vi "DAQmx Create Channel (TEDS-AI-Bridge).vi"(0 "task in":refnum<k21>, 1 "maximum value":dbl=0.002 format="%.3f", 2 "minimum value":dbl=-0.002 format="%.3f", 5 "physical channels":tag, 7 "name to assign":string, 9 "units":i32(ring)=12516 items=["From TEDS"=12516, "From Custom Scale"=10065], 11 "error in":errorcluster, 12 "custom scale name":tag, 13 "voltage excitation source":i32(ring)=10200 items=["Internal"=10200, "External"=10167], 14 "voltage excitation value":dbl=2.5) -> (4 "task out":refnum<k21>, 15 "error out":errorcluster)   [LabVIEW 2011]
doc: "Creates channel(s) that measure a Wheatstone bridge. You must configure the physical channel(s) with TEDS information to use this VI. Use this instance with bridge-based sensors that measure phenomena other than strain, force, pressure, or torque, or that scale data to physical units NI-DAQmx does not support."
uses:
  C:/Program Files/National Instruments/LabVIEW 2011/resource/objmgr/daqmx.rc
panel:
  # "input limits"
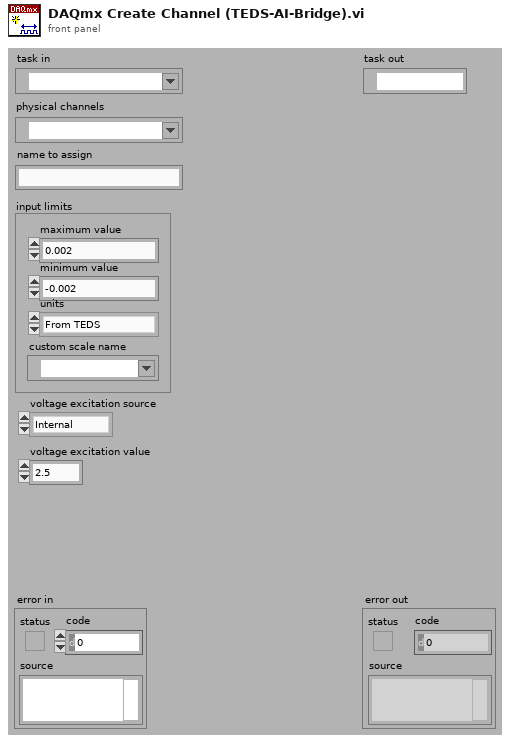
[diagram p1: front panel]
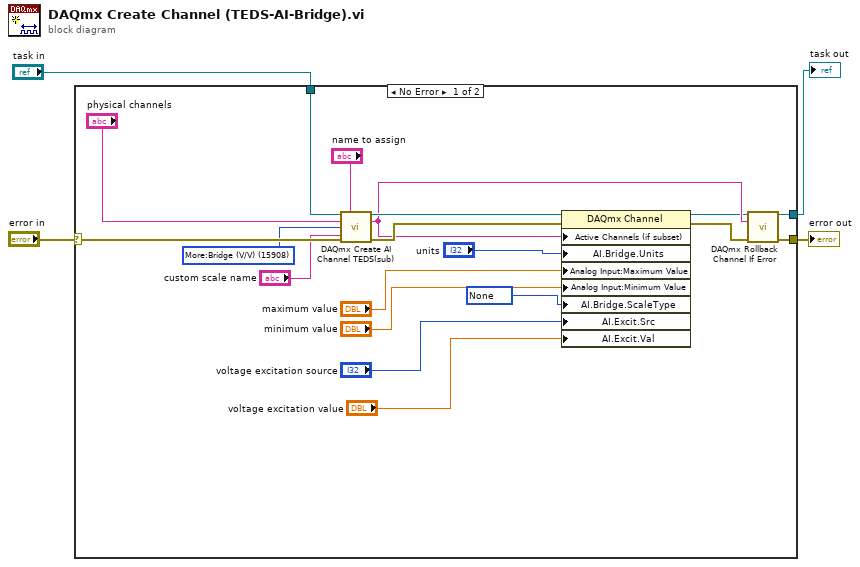
[diagram p0: block diagram]
diagram:
  n1 = case shown="No Error" "error in" {
    selector: "error in" -> [w22 w24]
    tunnel: [w14 w24] -> w4
    tunnel: "task in" -> [w23 w25]
    tunnel: [w13 w25] -> w1
    frame No Error {
      w8 = 10230 items=["None"=10230, "Two-Point Linear"=15898, "Table"=10450, "Polynomial"=10449] ("AI.Bridge.ScaleType")
      w9 = 15908 items=["Voltage"=10322, "Voltage RMS"=10350, "Current"=10134, "Current RMS"=10351, "More:Voltage:Custom with Excitation"=10323, "More:Bridge (V/V)"=15908, "Frequency"=10181, "Resistance"=10278, "Temperature:Thermocouple"=10303, "Temperature:Thermistor"=10302, "Temperature:RTD"=10301, "Temperature:Built-in Sensor"=10311, "Strain Gage"=10300, "Position:LVDT"=10352, "Position:RVDT"=10353, "Position:Eddy Current Proximity Probe"=14835, "Accelerometer"=10356, "Force:Bridge (Two-Point Linear)"=15899, "Force:Bridge (Table)"=15900, "Force:Bridge (Polynomial)"=15901, "Force:IEPE Sensor"=15895, "Pressure:Bridge (Two-Point Linear)"=15902, "Pressure:Bridge (Table)"=15903, "Pressure:Bridge (Polynomial)"=15904, "Sound Pressure:Microphone"=10354, "Torque:Bridge (Two-Point Linear)"=15905, "Torque:Bridge (Table)"=15906, "Torque:Bridge (Polynomial)"=15907, "TEDS Sensor"=12531] ("AI.MeasType")
      n2 = call "DAQmx Create AI Channel TEDS(sub).vi"("task in"=w23, "virtual channel name"="name to assign", "physical channel name"="physical channels", "measurement type"=w9, "error in"=w22, "custom scale"="custom scale name") -> ("task out"=w15:refnum<k21>, "channel names"=w12:string, "error out"=w20:errorcluster)  [unwired: 7 out]
      n3 = property class="DAQmx Channel"(reference=w15, error in=w20, "Active Channels (if subset)"=w12, "AI.Bridge.Units"="units", "Analog Input:Maximum Value"="maximum value", "Analog Input:Minimum Value"="minimum value", "AI.Bridge.ScaleType"=w8, "AI.Excit.Src"="voltage excitation source", "AI.Excit.Val"="voltage excitation value") -> (reference out=w11:refnum<k21>, error out=w10:errorcluster)
      n4 = call "DAQmx Rollback Channel If Error.vi"("task in"=w11, "channel names"=w12, "error in"=w10) -> ("task out"=w13:refnum<k21>, "error out"=w14:errorcluster)  [unwired: 11 out]
    }
    frame Error {
    }
  }
  "error out" <- w4
  "task out" <- w1
